vi "TcA04-001_DynamicallyCallSubClassMethods.vi"(1 "Input buffer":T3="1", 3 "Invocation info":T2, 5 "error in (no error)":errorcluster, 6 "Add log to result?":bool) -> (16 "Test Data":T1 {"Numeric Measurement" format="%.2f"}, 19 "error out":errorcluster)   [LabVIEW 2009]
doc: "Test case template."
uses:
  Shared/Support_InputBuffer.ctl
  Shared/Support_InvocationInfo.ctl
  Shared/Support_TestData.ctl
  TestClasses/G#BaseClass1_class/G#BaseClass1.lvclass
  TestClasses/G#SubClass1_class/G#SubClass1.lvclass
  TestClasses/G#SubSubClass1_class/G#SubSubClass1.lvclass
  <vilib>/addons/_AddQ/G#Object/G#Object.lvclass
panel:
  in  "Test name":string="TcA04-001 Dynamically call sub class methods"
  out "Test result":bool
  out "Result":string
  # "Verify that a sub class method can be dynamically called\n(if there exists one) by a virtually declared base \nclass method else base class implementation is used."
  # "Sub test case"
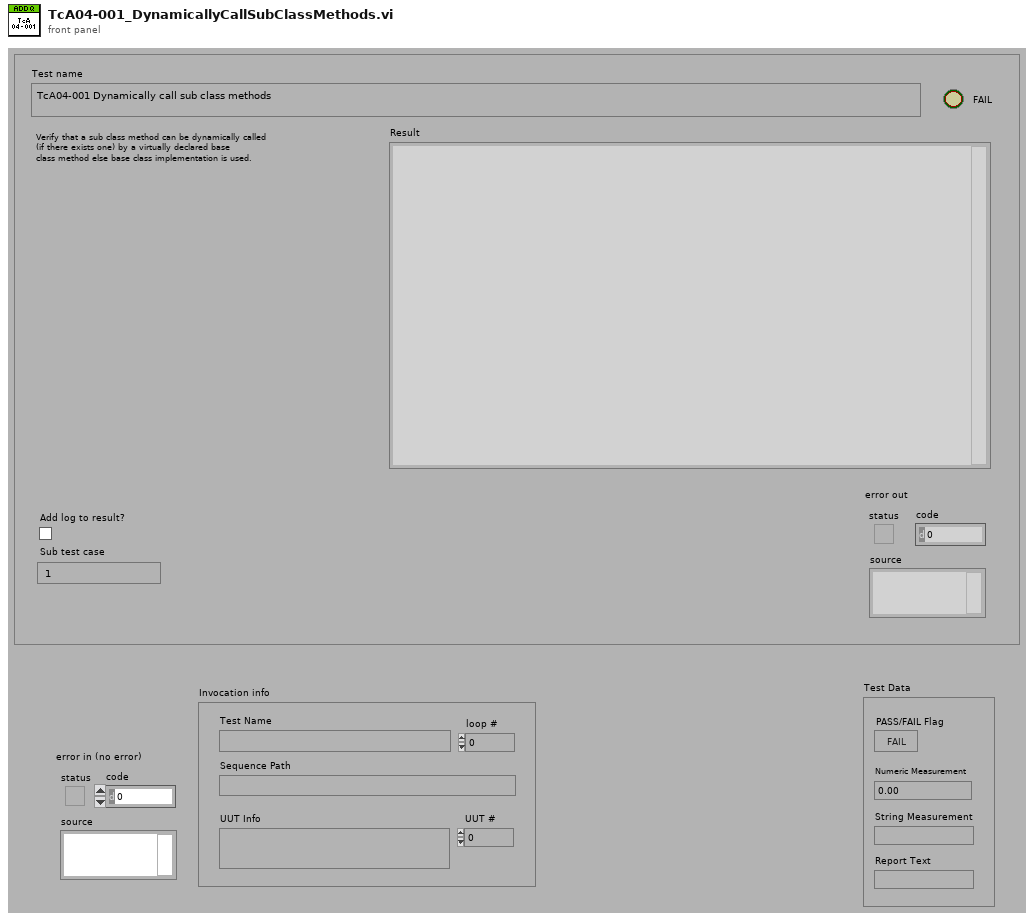
[diagram p1: front panel]
types:
  T1 = typedef "Support_TestData.ctl" = cluster{"PASS/FAIL Flag":bool, "Numeric Measurement":dbl, "String Measurement":string, "Report Text":string}
  T2 = typedef "Support_InvocationInfo.ctl" = cluster{"UUT #":i32, "loop #":i32, "UUT Info":string, "Test Name":string, "Sequence Path":path}
  T3 = typedef "Support_InputBuffer.ctl" = string
  T4 = typedef "Support_ResultType.ctl" = cluster{"Pass":bool, "Comment":string, "MeasurementValue":dbl}
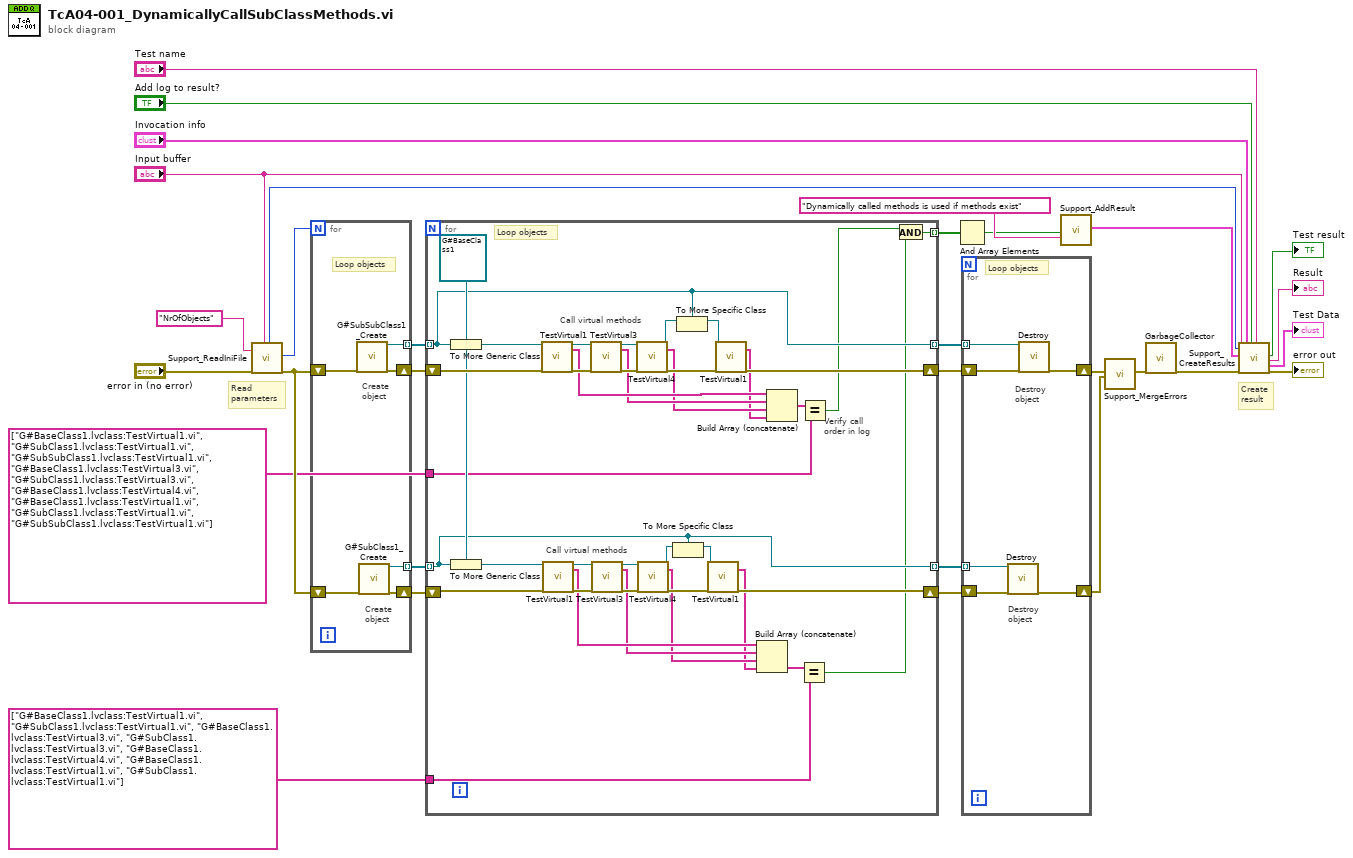
[diagram p0: block diagram]
diagram:
  # "Create\nresult"
  # "Read\nparameters"
  n1 = call "Support_ReadIniFile.vi"("Parameter name"="NrOfObjects", "error in (no error)"="error in (no error)", "Sub test case"="Input buffer") -> ("Timer start"=w21:u32, "Parameter1 as I32"=w18:i32, "error out"=w8:errorcluster)  [unwired: 9 in, 5 out]
  n2 = for {
    N: w18 -> [_]
    tunnel: [w37] -> w15 mode=indexing
    shift-right: [w36] -> w16
    shift-left: w8 -> [w35]
    shift-right: [w33] -> w6
    shift-left: w8 -> [w34]
    tunnel: [w32] -> w7 mode=indexing
    # "Create\nobject"
    # "Loop objects"
    # "Create\nobject"
    n3 = call "G#SubSubClass1_Create.vi"("error in (no error)"=w35) -> ("reference out"=w37:refnum<class "G#SubSubClass1.lvclass">, "error out"=w36:errorcluster)  [unwired: 17 in]
    n4 = call "G#SubClass1_Create.vi"("error in (no error)"=w34) -> ("reference out"=w32:refnum<class "G#SubClass1.lvclass">, "error out"=w33:errorcluster)  [unwired: 16 in, 1 out]
  }
  n5 = for {
    shift-right: [w67] -> w14
    shift-left: w16 -> [w74]
    tunnel: w15 -> [w69] mode=indexing
    tunnel: [w69] -> w13 mode=indexing
    tunnel: [w75] -> w12 mode=indexing
    tunnel: w7 -> [w68] mode=indexing
    shift-right: [w66] -> w4
    shift-left: w6 -> [w73]
    tunnel: [w68] -> w5 mode=indexing
    tunnel: string[] ["G#BaseClass1.lvclass:TestVirtual1.vi", "G#SubClass1.lvclass:TestVirtual1.vi", "G#SubSubClass1.lvclass:TestVirtual1.vi", "G#BaseClass1.lvclass:TestVirtual3.vi", "G#SubClass1.lvclass:TestVirtual3.vi", "G#BaseClass1.lvclass:TestVirtual4.vi", "G#BaseClass1.lvclass:TestVirtual1.vi", "G#SubClass1.lvclass:TestVirtual1.vi", "G#SubSubClass1.lvclass:TestVirtual1.vi"] ("appended array") -> [w41]
    tunnel: string[] ["G#BaseClass1.lvclass:TestVirtual1.vi", "G#SubClass1.lvclass:TestVirtual1.vi", "G#BaseClass1.lvclass:TestVirtual3.vi", "G#SubClass1.lvclass:TestVirtual3.vi", "G#BaseClass1.lvclass:TestVirtual4.vi", "G#BaseClass1.lvclass:TestVirtual1.vi", "G#SubClass1.lvclass:TestVirtual1.vi"] ("appended array 2") -> [w39]
    w70 = refnum<class "G#BaseClass1.lvclass"> refnum ("G#BaseClass1.lvclass")
    # "Call virtual methods"
    # "Call virtual methods"
    # "Loop objects"
    # "Verify call\norder in log"
    n6 = To More Generic Class(target class=w70, reference=w69) -> (generic class reference=w71:refnum<class "G#BaseClass1.lvclass">)
    n7 = To More Generic Class(target class=w70, reference=w68) -> (generic class reference=w72:refnum<class "G#BaseClass1.lvclass">)
    n8 = call-dynamic "TestVirtual1.vi"("reference in"=w71, "error in (no error)"=w74) -> ("reference out"=w62:refnum<class "G#BaseClass1.lvclass">, "MethodName"=w51:string[], "error out"=w65:errorcluster)  [unwired: 15 in]
    n9 = call-dynamic "TestVirtual1.vi"("reference in"=w72, "error in (no error)"=w73) -> ("reference out"=w57:refnum<class "G#BaseClass1.lvclass">, "MethodName"=w45:string[], "error out"=w56:errorcluster)  [unwired: 15 in]
    n10 = call-dynamic "TestVirtual3.vi"("reference in"=w62, "error in (no error)"=w65) -> ("reference out"=w61:refnum<class "G#BaseClass1.lvclass">, "MethodName"=w50:string[], "error out"=w64:errorcluster)  [unwired: 15 in]
    n11 = call-dynamic "TestVirtual3.vi"("reference in"=w57, "error in (no error)"=w56) -> ("reference out"=w58:refnum<class "G#BaseClass1.lvclass">, "MethodName"=w44:string[], "error out"=w55:errorcluster)  [unwired: 15 in]
    n12 = call-dynamic "TestVirtual4.vi"("reference in"=w61, "error in (no error)"=w64) -> ("reference out"=w60:refnum<class "G#BaseClass1.lvclass">, "MethodName"=w49:string[], "error out"=w63:errorcluster)  [unwired: 15 in]
    n13 = call-dynamic "TestVirtual4.vi"("reference in"=w58, "error in (no error)"=w55) -> ("reference out"=w53:refnum<class "G#BaseClass1.lvclass">, "MethodName"=w43:string[], "error out"=w54:errorcluster)  [unwired: 15 in]
    n14 = To More Specific Class(target class=w68, reference=w53) -> (specific class reference=w52:refnum<class "G#SubClass1.lvclass">)  [unwired: 1 in, 1 out]
    n15 = To More Specific Class(target class=w69, reference=w60) -> (specific class reference=w59:refnum<class "G#SubSubClass1.lvclass">)  [unwired: 1 in, 1 out]
    n16 = call-dynamic "TestVirtual1.vi"("reference in"=w52, "error in (no error)"=w54) -> ("MethodName"=w42:string[], "error out"=w66:errorcluster)  [unwired: 15 in, 1 out]
    n17 = call-dynamic "TestVirtual1.vi"("reference in"=w59, "error in (no error)"=w63) -> ("MethodName"=w46:string[], "error out"=w67:errorcluster)  [unwired: 15 in, 1 out]
    n18 = Build Array (concatenate)(w45, w44, w43, w42) -> (w40:string[])
    n19 = Build Array (concatenate)(w51, w50, w49, w46) -> (w48:string[])
    n20 = Equal?(x=w40, y=w39) -> (x = y?=w38:bool)
    n21 = Equal?(x=w48, y=w41) -> (x = y?=w47:bool)
    n22 = And(x=w47, y=w38) -> (x .and. y?=w75:bool)
  }
  n23 = And Array Elements(Boolean array=w12) -> (logical AND=w11:bool)
  n24 = for {
    shift-right: [w81] -> w9
    shift-left: w14 -> [w80]
    tunnel: w13 -> [w79] mode=indexing
    tunnel: w5 -> [w78] mode=indexing
    shift-right: [w76] -> w3
    shift-left: w4 -> [w77]
    # "Destroy\nobject"
    # "Loop objects"
    # "Destroy\nobject"
    n25 = call-dynamic "Destroy.vi"("reference in"=w78, "error in (no error)"=w77) -> ("error out"=w76:errorcluster)  [unwired: 16 in, 1 out]
    n26 = call-dynamic "Destroy.vi"("reference in"=w79, "error in (no error)"=w80) -> ("error out"=w81:errorcluster)  [unwired: 16 in, 1 out]
  }
  n27 = call "Support_AddResult.vi"("Pass"=w11, "Comment"="Dynamically called methods is used if methods exist") -> ("Results out"=w24:T4[])  [unwired: 17 in]
  n28 = call "Support_MergeErrors.vi"("error in 1"=w9, "error in 2"=w3) -> ("error out"=w10:errorcluster)  [unwired: 16 in, 1 out]
  n29 = call <vilib>:"GarbageCollector.vi"("error in (no error)"=w10) -> ("error out"=w20:errorcluster)  [unwired: 16 in, 2 out]
  n30 = call "Support_CreateResults.vi"("Sub test case"="Input buffer", "Timer start"=w21, "Results"=w24, "error in (no error)"=w20, "Invocation info"="Invocation info", "Add log to result?"="Add log to result?", "Test name"="Test name") -> ("Pass/fail flag"=→"Test result":bool, "Result"=→"Result":string, "Test Data"=→"Test Data":T1, "error out"=→"error out":errorcluster)  [unwired: 9 in]
